vi "Get Iteration.vi"(11 "Framework State in":refnum<class "Framework State.lvclass">) -> (2 "iteration":u64, 3 "Framework State out":refnum<class "Framework State.lvclass">)   [LabVIEW 2017, in "DSF Core.lvlib" / "Framework State.lvclass"]
uses:
  Framework State.lvclass
  Framework State.lvclass/Framework State.ctl
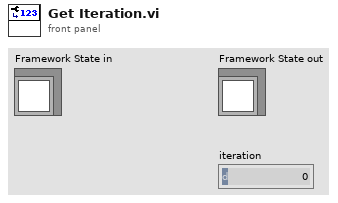
[diagram p1: front panel]
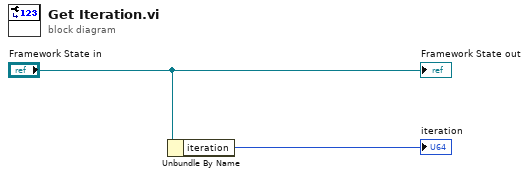
[diagram p0: block diagram]
diagram:
  n1 = Unbundle By Name("Framework State in") -> ("iteration"=→"iteration":u64)
  "Framework State out" <- "Framework State in"
